vi "DBC Sync Value To CAN Msg.vi"(9 "pCANMsg":u32, 10 "pMsgName":string, 11 "DBCHandle":cluster{}) -> (1 "pCANMsg out":u32, 2 "pMsgName out":string, 3 "function return":i32)   [LabVIEW 2010, in "dbc_parser.lvlib"]
doc: "int WINAPI DBC_SyncValueToCANMsg(long long DBCHandle, char* pMsgName, void* pCANMsg);"
uses:
  dbc_parser.lvlib
  USB2XXX/trunk/USB2XXX/USB2XXX/vs2019/Release/USB2XXX.dll
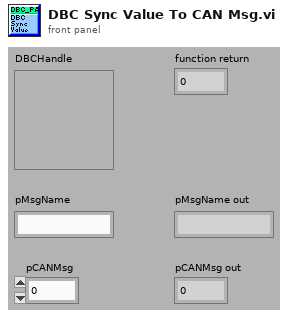
[diagram p1: front panel]
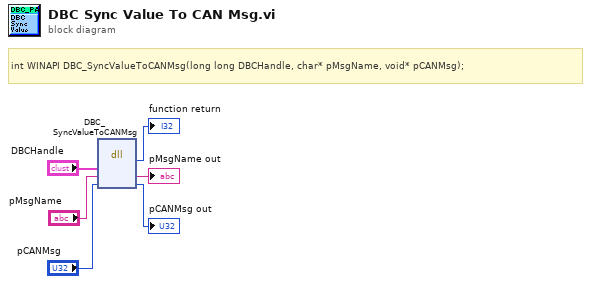
[diagram p0: block diagram]
diagram:
  # "int WINAPI DBC_SyncValueToCANMsg(long long DBCHandle, char* pMsgName, void* pCANMsg);"
  n1 = dll-call lib="E:/Projects/USB2XXX/trunk/USB2XXX/USB2XXX/vs2019/Release/USB2XXX.*" fn="DBC_SyncValueToCANMsg"("DBCHandle"="DBCHandle", "pMsgName"="pMsgName", "pCANMsg"="pCANMsg") -> (→"function return":i32, "pMsgName"=→"pMsgName out":string, "pCANMsg"=→"pCANMsg out":u32)  [unwired: 4 in, 2 out]
